vi "8.vi"(11 "文字列入力":string) -> (3 "文字列出力":string)   [LabVIEW 2019]
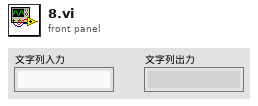
[diagram p1: front panel]
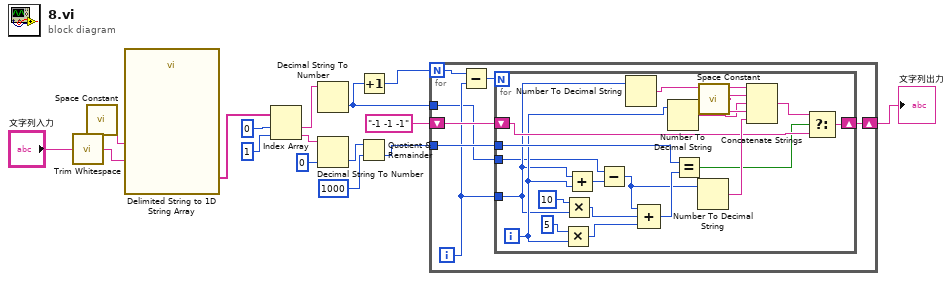
[diagram p0: block diagram]
diagram:
  n1 = call <vilib>:"Trim Whitespace.vi"("string"="文字列入力") -> ("trimmed string"=w5:string)  [unwired: 1 in]
  n2 = call <vilib>:"Space Constant.vi"() -> ("String"=w8:string)
  n3 = call <vilib>:"Delimited String to 1D String Array.vi"("delimiter"=w8, "delimited string"=w5) -> ("string array"=w11:string[])  [unwired: 9 in]
  n4 = Index Array ("指標配列")(array=w11, index #1=0, index #2=1) -> (element #1=w12:string, element #2=w7:string)
  n5 = Decimal String To Number(string=w12) -> (number=w2:i32)  [unwired: 2 in, 1 out]
  n6 = Decimal String To Number(string=w7, default (0L)=0 ("デフォルト (0 I32)")) -> (number=w3:i32)  [unwired: 1 in, 1 out]
  n7 = Increment(x=w2) -> (x+1=w13:i32)
  n8 = Quotient & Remainder(x=w3, y=1000) -> (floor(x/y)=w6:i32)  [unwired: 1 out]
  n9 = for {
    N: w13 -> [w23]
    tunnel: w6 -> [w21]
    shift-right: [w18] -> w15
    shift-left: "-1 -1 -1" -> [w20]
    tunnel: w2 -> [w17]
    i -> [w19]
    n10 = Subtract(x=w23, y=w19) -> (x-y=w22:i32)
    n11 = for {
      N: w22 -> [_]
      tunnel: w21 -> [w40]
      tunnel: w19 -> [w28]
      shift-right: [w39] -> w18
      shift-left: w20 -> [w35]
      tunnel: w17 -> [w27]
      i -> [w29]
      n12 = Multiply(x=5, y=w29) -> (x*y=w32:i32)
      n13 = Multiply(x=10, y=w28) -> (x*y=w33:i32)
      n14 = Add(x=w28, y=w29) -> (x+y=w26:i32)
      n15 = Subtract(x=w27, y=w26) -> (x-y=w25:i32)
      n16 = Number To Decimal String(number=w28) -> (decimal integer string=w38:string)  [unwired: 1 in]
      n17 = Compound Arithmetic op=ADD(w25, w33, w32) -> (w31:i32)
      n18 = Number To Decimal String(number=w29) -> (decimal integer string=w24:string)  [unwired: 1 in]
      n19 = Equal?(x=w40, y=w31) -> (x = y?=w30:bool)
      n20 = Number To Decimal String(number=w25) -> (decimal integer string=w36:string)  [unwired: 1 in]
      n21 = call <vilib>:"Space Constant.vi"() -> ("String"=w37:string)
      n22 = Concatenate Strings(w38, w37, w24, w37, w36) -> (w34:string)
      n23 = Select(t=w34, s=w30, f=w35) -> (s? t:f=w39:string)
    }
  }
  "文字列出力" <- w15
